vi "draw rotated rectangle.vi"(4 "fill":bool, 5 "Color Box":u32(colorbox), 6 "angle":dbl, 7 "2D Picture":picture, 8 "height":dbl, 9 "width":dbl, 10 "y":dbl, 11 "x":dbl) -> (3 "new picture":picture)   [LabVIEW 2021]
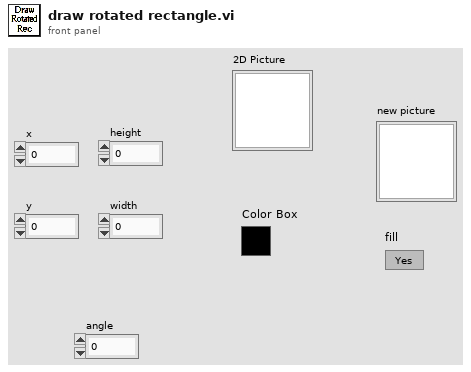
[diagram p1: front panel]
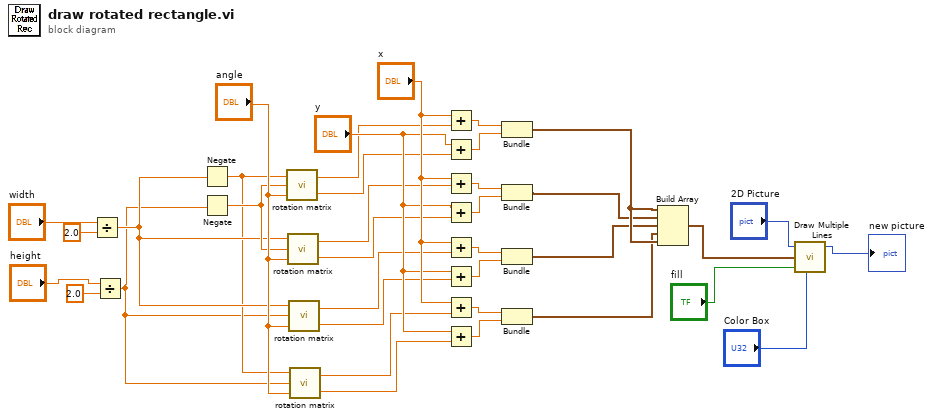
[diagram p0: block diagram]
diagram:
  n1 = Divide(x="width", y=2.0) -> (x/y=w4:dbl)
  n2 = Divide(x="height", y=2.0) -> (x/y=w2:dbl)
  n3 = Negate(x=w4) -> (-x=w3:dbl)
  n4 = Negate(x=w2) -> (-x=w5:dbl)
  n5 = call "rotation matrix.vi"("angle"="angle", "y"=w5, "x"=w3) -> ("new y"=w12:dbl, "new x"=w13:dbl)
  n6 = call "rotation matrix.vi"("angle"="angle", "y"=w5, "x"=w4) -> ("new y"=w10:dbl, "new x"=w11:dbl)
  n7 = call "rotation matrix.vi"("angle"="angle", "y"=w2, "x"=w4) -> ("new y"=w8:dbl, "new x"=w9:dbl)
  n8 = call "rotation matrix.vi"("angle"="angle", "y"=w2, "x"=w3) -> ("new y"=w6:dbl, "new x"=w7:dbl)
  n9 = Add(x="x", y=w13) -> (x+y=w21:dbl)
  n10 = Add(x="y", y=w12) -> (x+y=w22:dbl)
  n11 = Add(x="x", y=w11) -> (x+y=w23:dbl)
  n12 = Add(x="y", y=w10) -> (x+y=w24:dbl)
  n13 = Add(x="x", y=w9) -> (x+y=w25:dbl)
  n14 = Add(x="y", y=w8) -> (x+y=w26:dbl)
  n15 = Add(x="x", y=w7) -> (x+y=w27:dbl)
  n16 = Add(x="y", y=w6) -> (x+y=w28:dbl)
  n17 = Bundle(w21, w22) -> (w20:cluster{dbl, dbl})  [unwired: 1 in]
  n18 = Bundle(w23, w24) -> (w19:cluster{dbl, dbl})  [unwired: 1 in]
  n19 = Bundle(w25, w26) -> (w18:cluster{dbl, dbl})  [unwired: 1 in]
  n20 = Bundle(w27, w28) -> (w17:cluster{dbl, dbl})  [unwired: 1 in]
  n21 = Build Array(w20, w19, w18, w17, w20) -> (w35:cluster{dbl, dbl}[])
  n22 = call <vilib>:"Draw Multiple Lines.vi"("picture"="2D Picture", "line endpoints"=w35, "fill?(F)"="fill", "color(black)"="Color Box") -> ("new picture"=→"new picture":picture)  [unwired: 5 in]
